vi "运维调试.vi"() -> ()   [LabVIEW 2016]
uses:
  <vilib>/Utility/miscctls.llb/LVPointTypeDef.ctl
panel:
  in  "运维调试单选按钮":enum32{"营养盐", "CodMn", "总磷总氮", "多参数", "其他"}(xcontrol)
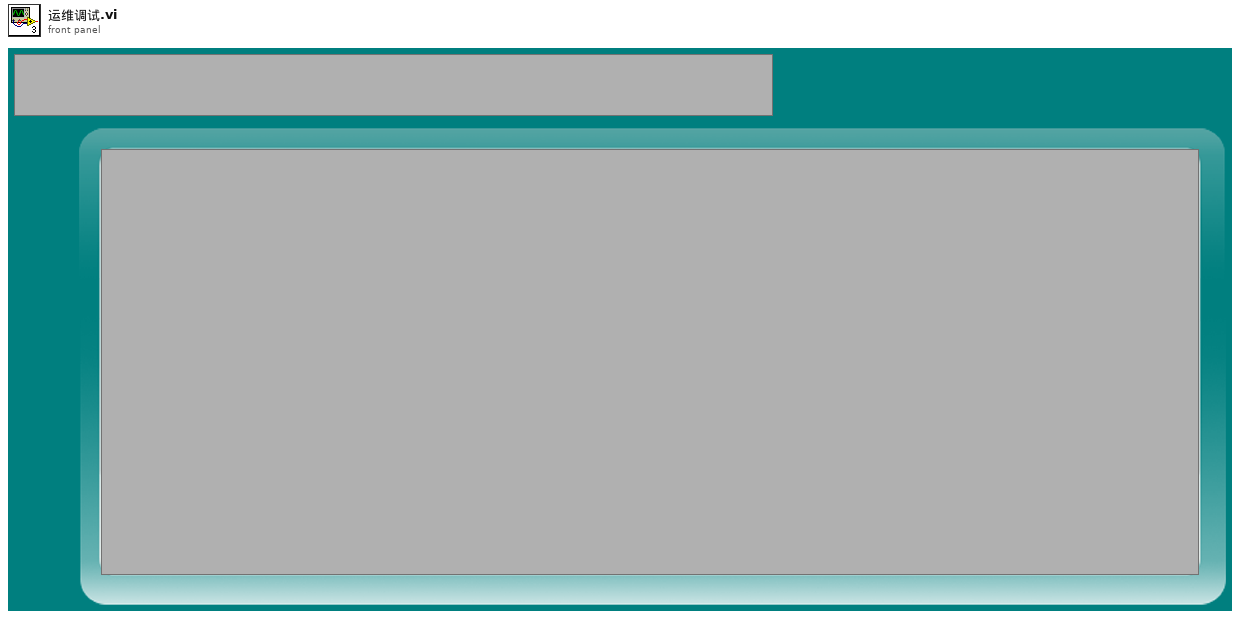
[diagram p1: front panel]
types:
  T1 = typedef "LVPointTypeDef.ctl" = cluster{"Horizontal":i16, "Vertical":i16}
  T2 = enum32{"Bad", "Idle", "Run top level", "Running"}
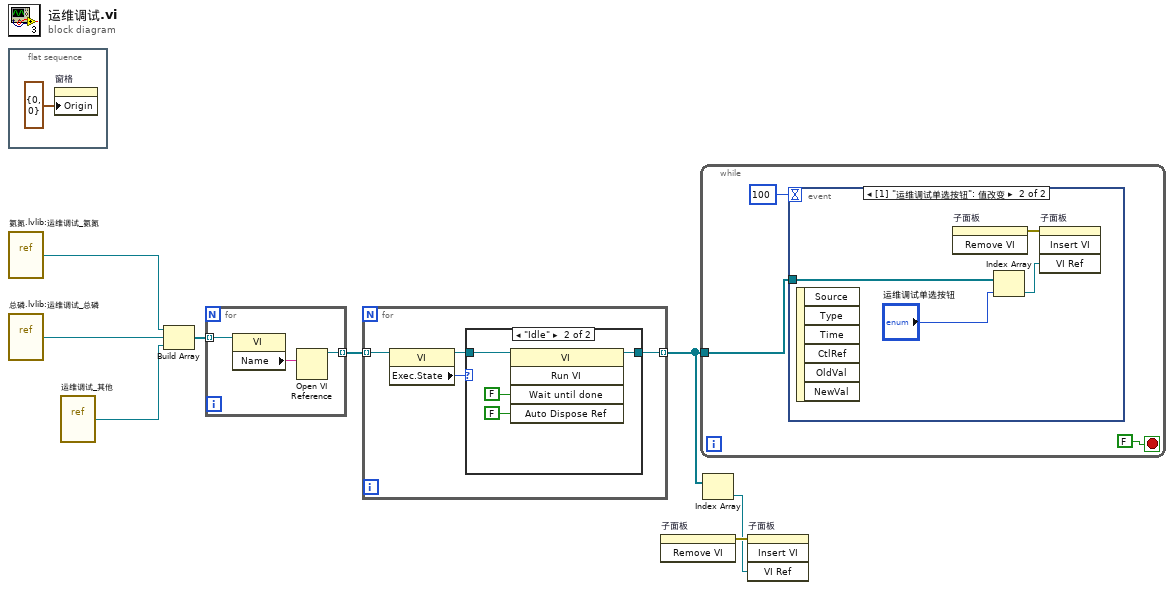
[diagram p0: block diagram]
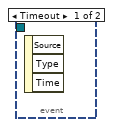
[diagram p3: hidden frame]
diagram:
  n1 = flat-sequence {
    frame #0 {
      n2 = property on="窗格" class="Pane"("Origin"=T1 {"Horizontal"=0, "Vertical"=0} ("原点")) -> ()  [unwired: 2 in, 2 out]
    }
  }
  n3 = vi-ref "氨氮.lvlib:运维调试_氨氮.vi"() -> (w4:refnum<vi>)
  n4 = vi-ref "总磷.lvlib:运维调试_总磷.vi"() -> (w2:refnum<vi>)
  n5 = vi-ref "运维调试_其他.vi"() -> (w1:refnum<vi>)
  n6 = Build Array(w4, w2, w1) -> (w3:refnum<vi>[])
  n7 = for {
    tunnel: [w12] -> w8 mode=indexing
    tunnel: w3 -> [w11] mode=indexing
    n8 = property class="VI"(reference=w11) -> ("Name"=w10:string)  [unwired: 1 in, 2 out]
    n9 = Open VI Reference(vi path=w10) -> (vi reference=w12:refnum<vi>)  [unwired: 5 in, 1 out]
  }
  n10 = for {
    tunnel: w8 -> [w16] mode=indexing
    tunnel: [w13] -> w6 mode=indexing
    n11 = property class="VI"(reference=w16) -> (reference out=w14:refnum<vi>, "Exec.State"=w15:T2)  [unwired: 1 in, 1 out]
    n12 = case shown="\"Idle\"" w15 {
      tunnel: w14 -> [w17 w19]
      tunnel: [w17 w18] -> w13
      frame "Bad", Default {
      }
      frame "Idle" {
        n13 = invoke class="VI" method="Run VI"(reference=w19, "Wait until done"=FALSE ("结束前等待"), "Auto Dispose Ref"=FALSE ("自动销毁引用")) -> (reference out=w18:refnum<vi>)  [unwired: 2 in, 4 out]
      }
    }
  }
  n14 = invoke on="子面板" class="SubPnl" method="Remove VI"() -> (error out=w7:errorcluster)  [unwired: 3 in, 2 out]
  n15 = while {
    tunnel: w6 -> [w23]
    stop <- FALSE stop-if-true
    n16 = event shown="[1] \"运维调试单选按钮\": 值改变" {
      selector: _ -> [_ _]
      dyn-events: _ -> [_ _]
      timeout: 100 -> [_ _]
      tunnel: w23 -> [_ w26]
      event Timeout {
        n17 = event-data() -> ()  [unwired: 1 in, 3 out]
      }
      event "运维调试单选按钮": Value Change {
        n18 = event-data() -> ()  [unwired: 1 in, 6 out]
        n19 = invoke on="子面板" class="SubPnl" method="Remove VI"() -> (error out=w28:errorcluster)  [unwired: 3 in, 2 out]
        n20 = Index Array(array=w26, index="运维调试单选按钮") -> (element=w25:refnum<vi>)
        n21 = invoke on="子面板" class="SubPnl" method="Insert VI"(error in=w28, "VI Ref"=w25) -> ()  [unwired: 2 in, 4 out]
      }
    }
  }
  n22 = Index Array(array=w6) -> (element=w5:refnum<vi>)  [unwired: 1 in]
  n23 = invoke on="子面板" class="SubPnl" method="Insert VI"(error in=w7, "VI Ref"=w5) -> ()  [unwired: 2 in, 4 out]
